vi "Digital Input - N Channels - N Samples.vi"() -> ()   [LabVIEW 2019]
uses:
  <vilib>/myRIO/Common/Instrument Driver Framework/ELVIS III v1.0/DI Block/vis/ELVIS III v1.0 DI Block Read.vi
  <vilib>/myRIO/Common/Instrument Driver Framework/ELVIS III v1.0/DI Block/vis/ELVIS III v1.0 Close DI Block.vi
  <vilib>/myRIO/Common/Instrument Driver Framework/myRIO v1.0/UART/vis/myRIO v1.0 Close UART.vi
  <vilib>/myRIO/Common/Instrument Driver Framework/Utilities/vis/Sample Rate To Ticks.vi
  <vilib>/myRIO/Common/Instrument Driver Framework/ELVIS III v1.0/DI Block/vis/ELVIS III v1.0 Unreserve DI Block.vi
  <vilib>/myRIO/Common/Instrument Driver Framework/ELVIS III v1.0/DI Block/vis/ELVIS III v1.0 Build MUX Configuration DI Block.vi
  <vilib>/myRIO/Common/Instrument Driver Framework/ELVIS III v1.0/Resource Manager/vis/ELVIS III v1.0 Create Configuration List.vi
  <vilib>/Utility/error.llb/Error Cluster From Error Code.vi
  <vilib>/myRIO/Common/Instrument Driver Framework/myRIO v1.0/Resource Manager/vis/myRIO v1.0 Block Write Configuration.vi
  <vilib>/myRIO/Common/Instrument Driver Framework/ELVIS III v1.0/DI Block/vis/ELVIS III v1.0 DI Block Read Bank B.vi
  <vilib>/myRIO/Common/Instrument Driver Framework/ELVIS III v1.0/DI Block/vis/ELVIS III v1.0 DI Block Read Bank A.vi
  <vilib>/Waveform/DWDTOps.llb/DWDT Boolean Array to Digital.vi
  <vilib>/myRIO/Common/Instrument Driver Framework/ELVIS III v1.0/Resource Manager/vis/ELVIS III v1.0 Configure IO.vi
  <vilib>/myRIO/Common/Instrument Driver Framework/ELVIS III v1.0/Resource Manager/vis/ELVIS III v1.0 Configure DI Mode.vi
  <vilib>/myRIO/Common/Instrument Driver Framework/ELVIS III v1.0/Resource Manager/vis/ELVIS III v1.0 Unreserve Channel List.vi
  <vilib>/myRIO/Common/Instrument Driver Framework/myRIO v1.0/myRIO v1.0 Close.vi
  <vilib>/myRIO/Common/Instrument Driver Framework/Utilities/vis/FPGA Ref Manager.vi
  <vilib>/myRIO/Common/Instrument Driver Framework/ELVIS III v1.0/ELVIS III v1.0 Reset FPGA.vi
  <vilib>/myRIO/Common/Instrument Driver Framework/myRIO v1.0/IRQ/vis/myRIO v1.0 IRQ Info FGV.vi
  <vilib>/myRIO/Common/Instrument Driver Framework/myRIO v1.0/IRQ/vis/myRIO v1.0 Timer IRQ Info FGV.vi
  <vilib>/myRIO/Common/Instrument Driver Framework/myRIO v1.0/IRQ/vis/myRIO v1.0 ISR Agent.vi
  <vilib>/myRIO/Instrument Drivers/Utilities/vis/Reset Index.vi
  <vilib>/myRIO/Common/Instrument Driver Framework/myRIO v1.0/Resource Manager/vis/myRIO v1.0 Block Write Resource Manager.vi
  <vilib>/myRIO/Instrument Drivers/Utilities/Utilities.lvlib
  <vilib>/myRIO/Instrument Drivers/Onboard IO/DI Block/DI Block.lvlib
panel:
  in  "Acquire Data":bool
  in  "Stop":bool
  out "Digital Waveform Graph":digitalwaveform(graph)
  # "ELVIS III Control IO"
  # "数字输入N通道"
  # "Overview: Acquires N sample digital data on Bank A, Channels 0 and 1 (A/DIO0 and A/DIO1).\nInstructions:\n1. Connect A/DIO0 and A/DIO1 to valid signals.\n2. Run the VI.\n3. Press Acquire Data to trigger a digital acquisition."
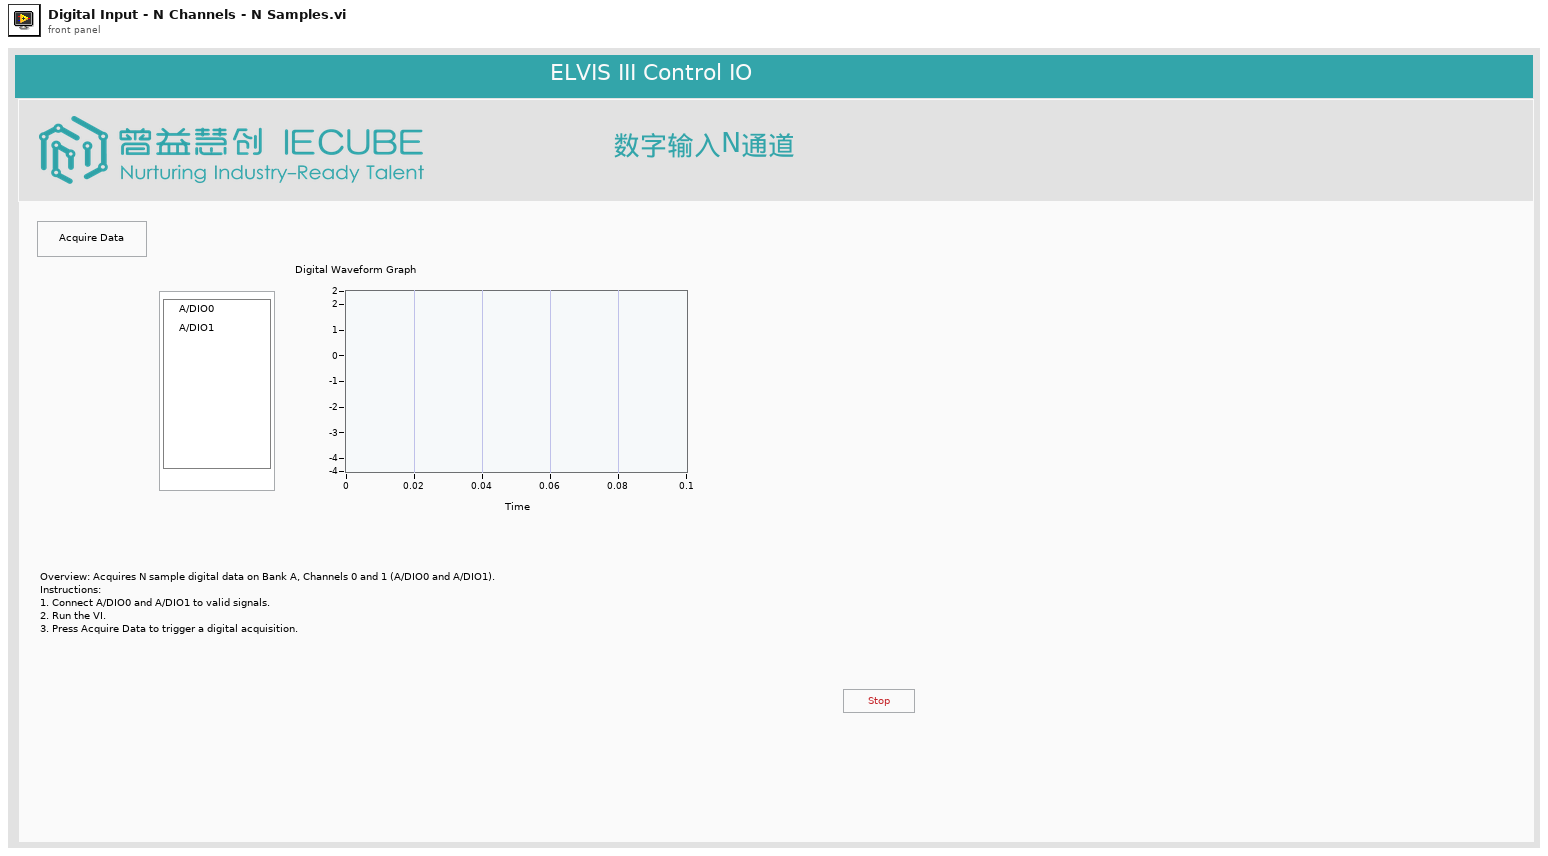
[diagram p1: front panel]
types:
  T1 = typedef "DI Block.lvlib/DI Block Reference.ctl" = cluster{"myRIO Reference":T2, "DI (N Samples) Channels List":T6}
  T2 = typedef "myRIO Generic Hardware Reference.ctl" = cluster{"myRIO Model":T3, "myRIO Hardware Reference":T4}
  T3 = typedef "Hardware Version Enum.ctl" = enum16{"Unknown", "myRIO-1900", "myRIO-1950", "roboRIO", "NI ELVIS RIO CM", "ELVIS III"}
  T4 = typedef "myRIO v1.0 Reference.ctl" = cluster{"Generic FPGA Reference":T5, "Allow multiple opens":bool}
  T5 = typedef "Generic FPGA Reference.ctl" = refnum<k20>
  T6 = typedef "DI Block Channels List.ctl" = T7[]
  T7 = typedef "DI Block Channels Enum.ctl" = enum16{"Not Connected", "A/DI0 (N Samples)", "A/DI1 (N Samples)", "A/DI2 (N Samples)", "A/DI3 (N Samples)", "A/DI4 (N Samples)", "A/DI5 (N Samples)", "A/DI6 (N Samples)", "A/DI7 (N Samples)", "A/DI8 (N Samples)", "A/DI9 (N Samples)", "A/DI10 (N Samples)", "A/DI11 (N Samples)", "A/DI12 (N Samples)", "A/DI13 (N Samples)", "A/DI14 (N Samples)", "A/DI15 (N Samples)", "A/DI16 (N Samples)", "A/DI17 (N Samples)", "A/DI18 (N Samples)", "A/DI19 (N Samples)", "B/DI0 (N Samples)", "B/DI1 (N Samples)", "B/DI2 (N Samples)", "B/DI3 (N Samples)", "B/DI4 (N Samples)", "B/DI5 (N Samples)", "B/DI6 (N Samples)", "B/DI7 (N Samples)", "B/DI8 (N Samples)", "B/DI9 (N Samples)", "B/DI10 (N Samples)", "B/DI11 (N Samples)", "B/DI12 (N Samples)", "B/DI13 (N Samples)", "B/DI14 (N Samples)", "B/DI15 (N Samples)", "B/DI16 (N Samples)", "B/DI17 (N Samples)", "B/DI18 (N Samples)", "B/DI19 (N Samples)"}
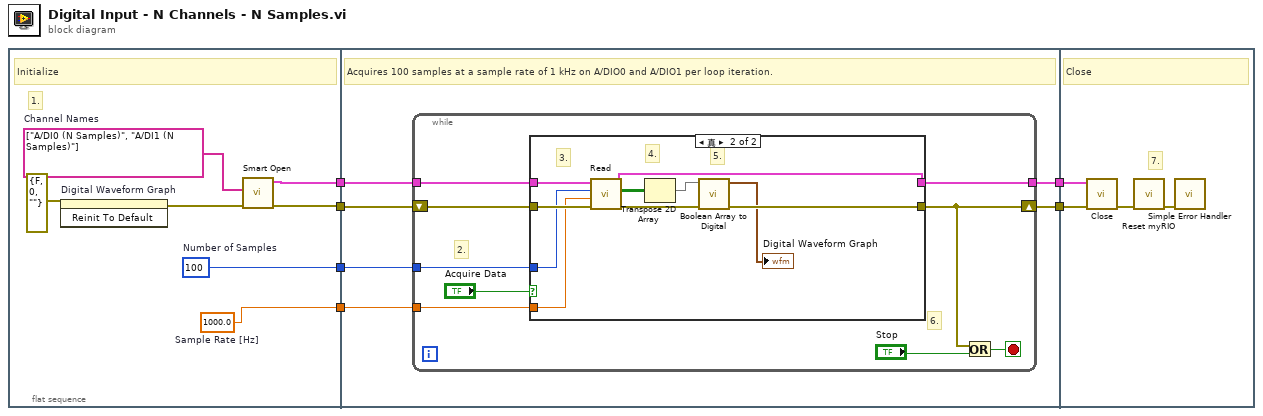
[diagram p0: block diagram]
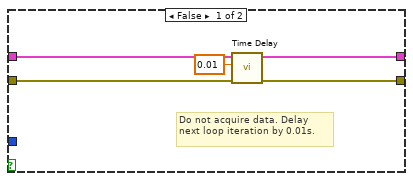
[diagram p2: hidden frame]
diagram:
  n1 = flat-sequence {
    tunnel: [w10] -> w5
    tunnel: [w9] -> w4
    tunnel: [w8] -> w3
    tunnel: [w7] -> w2
    tunnel: [w19] -> w6
    tunnel: w5 -> [w18]
    tunnel: w4 -> [w17]
    tunnel: w3 -> [w16]
    tunnel: w2 -> [w15]
    tunnel: [w14] -> w1
    tunnel: w6 -> [w45]
    tunnel: w1 -> [w43]
    frame #0 {
      w7 = 1000.0  # Sample Rate [Hz]
      w8 = u32 100  # Number of Samples
      w12 = tag[] ["A/DI0 (N Samples)", "A/DI1 (N Samples)"]  # Channel Names
      # "1."
      # "Initialize"
      n2 = invoke on="Digital Waveform Graph" class="DigitalGraph (strict)" method="Reinit To Default"(error in=errorcluster {"status"=FALSE, "code"=0, "source"=""} ("Error In")) -> (error out=w11:errorcluster)  [unwired: 2 in, 2 out]
      n3 = call <vilib>:"Smart Open.vi"("error in (no error)"=w11, "Channel Names"=w12) -> ("error out"=w10:errorcluster, "DI (N Samples) Ref Out"=w9:T1)  [unwired: 8 in]
    }
    frame #1 {
      # "Acquires 100 samples at a sample rate of 1 kHz on A/DIO0 and A/DIO1 per loop iteration."
      n4 = while {
        shift-right: [w26] -> w19
        shift-left: w18 -> [w27]
        tunnel: w17 -> [w23]
        tunnel: w16 -> [w22]
        tunnel: w15 -> [w21]
        tunnel: [w20] -> w14
        stop <- w28 stop-if-true
        # "6."
        # "2."
        n5 = case shown="真" "Acquire Data" {
          tunnel: w27 -> [w31 w40]
          tunnel: [w30 w42] -> w26
          tunnel: w23 -> [w29 w37]
          tunnel: w22 -> [_ w36]
          tunnel: w21 -> [_ w35]
          tunnel: [w29 w34] -> w20
          frame False {
            # "Do not acquire data. Delay next loop iteration by 0.01s."
            n6 = call "Time Delay"("error in (no error)"=w31, "Delay Time (s)"=0.01) -> ("error out"=w30:errorcluster)  [unwired: 9 in]
          }
          frame True {
            # "5."
            # "4."
            # "3."
            n7 = call <vilib>:"Read.vi"("error in (no error)"=w40, "Sample Rate [Hz]"=w35, "Number of Samples"=w36, "DI (N Samples) Ref In"=w37) -> ("error out"=w38:errorcluster, "Values"=w39:bool[][], "DI (N Samples) Ref Out"=w34:T1)  [unwired: 5 in]
            n8 = Transpose 2D Array(2D array=w39) -> (transposed array=w41:bool[][])
            n9 = call-poly <vilib>:"Boolean Array to Digital.vi"("error in (no error)"=w38, "boolean array"=w41) -> ("error out"=w42:errorcluster, "digital waveform"=→"Digital Waveform Graph":digitalwaveform)  [unwired: 8 in]
          }
        }
        n10 = Or(x=w26, y="Stop") -> (x .or. y?=w28:bool)
      }
    }
    frame #2 {
      # "7."
      # "Close"
      n11 = call <vilib>:"Close.vi"("error in (no error)"=w45, "DI (N Samples) Ref In"=w43) -> ("error out"=w44:errorcluster)  [unwired: 9 in]
      n12 = call <vilib>:"Reset myRIO.vi"("error in (no error)"=w44) -> ("error out"=w46:errorcluster)  [unwired: 10 in]
      n13 = call <vilib>:"Simple Error Handler.vi"("error in (no error)"=w46) -> ()  [unwired: 4 in, 5 out]
    }
  }
